vi "Registration_VI.vi"(8 "error in (no error)":errorcluster, 11 "Class 3 in":refnum<class "Panel3.lvclass">) -> (0 "error out":errorcluster, 2 "Core_Reference_VI out":refnum<vi>, 3 "Class 3 out":refnum<class "Panel3.lvclass">)   [LabVIEW 2021, in "Panel3.lvclass"]
uses:
  Panel3.lvclass
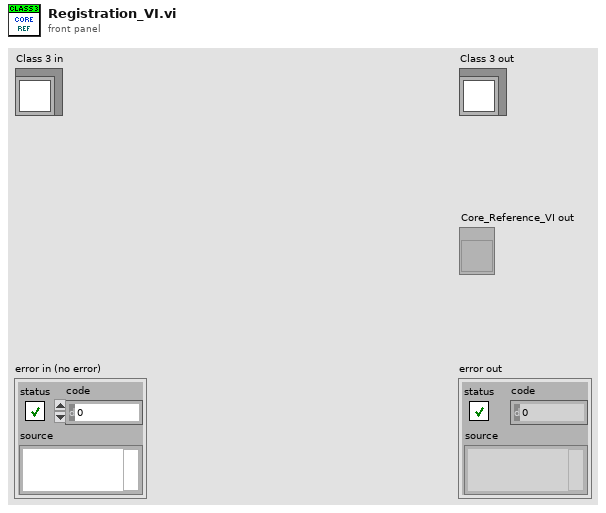
[diagram p1: front panel]
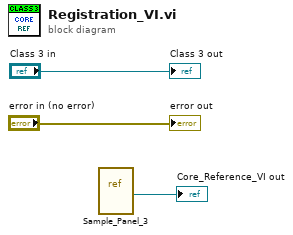
[diagram p0: block diagram]
diagram:
  n1 = vi-ref "Sample_Panel_3.vi"() -> (→"Core_Reference_VI out":refnum<vi>)
  "error out" <- "error in (no error)"
  "Class 3 out" <- "Class 3 in"
